vi "Read TCP Refnum.vi"(8 "error in (no error)":errorcluster, 11 "VISA TCP in":refnum<class "VISA TCP.lvclass">) -> (0 "error out":errorcluster, 2 "TCP Refnum":refnum<k5>, 3 "VISA TCP out":refnum<class "VISA TCP.lvclass">)   [LabVIEW 2021, in "Sockets.lvlib" / "VISA TCP.lvclass"]
doc: "WebSockets 2.0.1.40\nSam Sharp - MediaMongrels Ltd\nCopyright (c) 2019, MediaMongrels Ltd"
uses:
  VISA TCP.lvclass
  VISA TCP.lvclass/VISA TCP.ctl
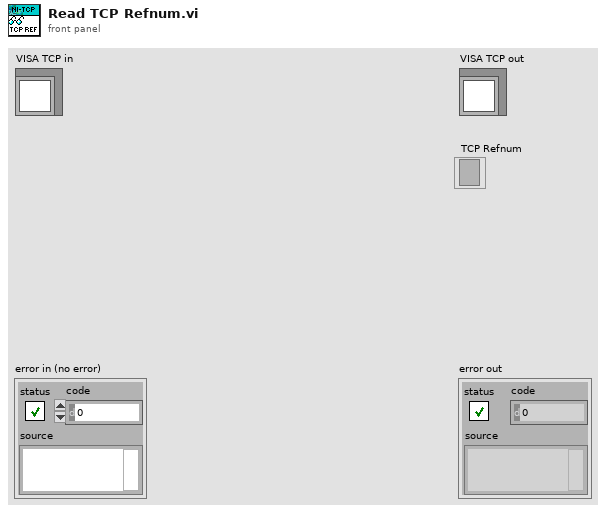
[diagram p1: front panel]
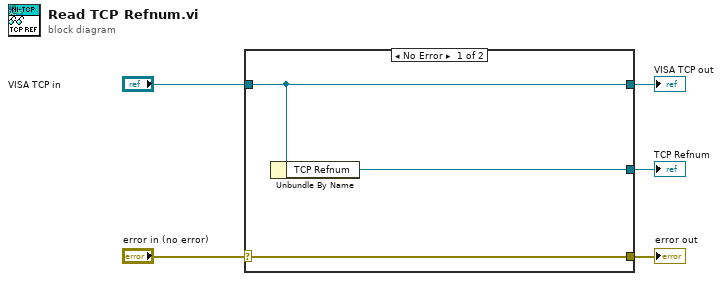
[diagram p0: block diagram]
diagram:
  n1 = case shown="No Error" "error in (no error)" {
    selector: "error in (no error)" -> [w8 w9]
    tunnel: [w8 w9] -> w4
    tunnel: [w7 w10] -> w2
    tunnel: "VISA TCP in" -> [w7 w10]
    tunnel: [w6 _] -> w1
    frame No Error {
      n2 = Unbundle By Name(w7) -> ("TCP Refnum"=w6:refnum<k5>)
    }
    frame Error {
    }
  }
  "error out" <- w4
  "VISA TCP out" <- w2
  "TCP Refnum" <- w1
